vi "Configure Average.vi"(7 "Average On (F)":bool, 8 "error in (no error)":errorcluster, 10 "Average":u32=1, 11 "MXA in":refnum<class "MXA.lvclass">) -> (0 "error out":errorcluster, 3 "MXA out":refnum<class "MXA.lvclass">)   [LabVIEW 2020, in "MXA.lvclass"]
uses:
  MXA.lvclass
  C:/Sandbox/RF Bench/Source Code/WiSpry Test Framework/Instruments/Instrument.lvclass
  Instrument.lvclass/Instrument.ctl
  Instrument.lvclass
  <instrlib>/Agilent MXA Series/Agilent MXA Series.lvlib
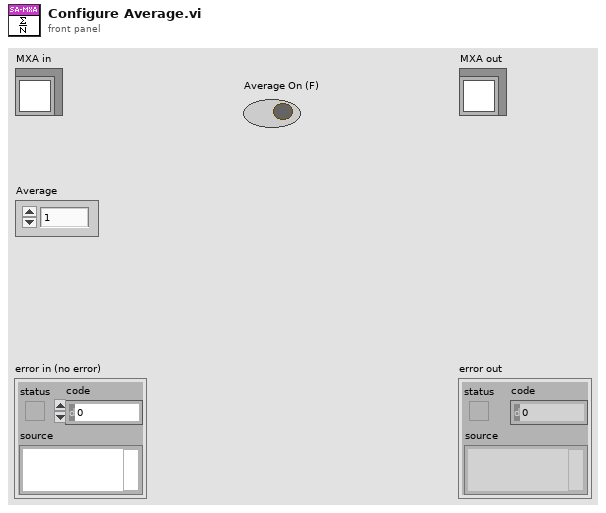
[diagram p1: front panel]
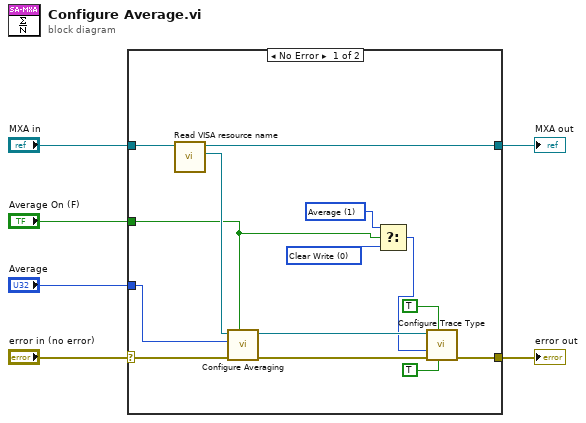
[diagram p0: block diagram]
diagram:
  n1 = case shown="No Error" "error in (no error)" {
    selector: "error in (no error)" -> [w16 w22]
    tunnel: "MXA in" -> [w20 w21]
    tunnel: [w14 w22] -> w6
    tunnel: [w19 w21] -> w5
    tunnel: "Average" -> [w17 _]
    tunnel: "Average On (F)" -> [w10 _]
    frame No Error {
      w8 = 0 items=["Clear Write", "Average", "Maximum Hold", "Minimum Hold"] ("Trace Type (0: Clear Write)")
      w9 = 1 items=["Clear Write", "Average", "Maximum Hold", "Minimum Hold"] ("Trace Type (0: Clear Write)")
      n2 = call "Read VISA resource name.vi"("Instrument in"=w20) -> ("VISA resource name"=w18:refnum<visa-resource-name>, "Instrument out"=w19:refnum<class "MXA.lvclass">)  [unwired: 9 in]
      n3 = call <instrlib>:"Configure Averaging.vi"("Enable Averaging (T: Enable)"=w10, "error in (no error)"=w16, "Average Count (100)"=w17, "VISA resource name"=w18) -> ("error out"=w15:errorcluster, "VISA resource name out"=w13:refnum<visa-resource-name>)  [unwired: 6 in]
      n4 = Select(t=w9, s=w10, f=w8) -> (s? t:f=w7:i32)
      n5 = call <instrlib>:"Configure Trace Type.vi"("Enable Trace Display (F: Disable)"=TRUE, "Enable Trace Update (F: Disable)"=TRUE, "error in (no error)"=w15, "Trace Type (0: Clear Write)"=w7, "VISA resource name"=w13) -> ("error out"=w14:errorcluster)  [unwired: 5 in, 1 out]
    }
    frame Error {
    }
  }
  "error out" <- w6
  "MXA out" <- w5
